vi "button painter (SubVI).vi"(9 "Off state":cluster{"accent color":u32, "accent color":u32}, 10 "On state":T1, 11 "Button ref in":refnum<vi>) -> ()   [LabVIEW 2021]
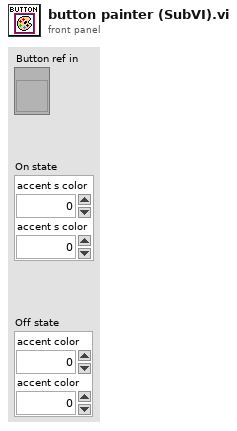
[diagram p1: front panel]
types:
  T1 = cluster{"accent s color":u32, "accent s color":u32}
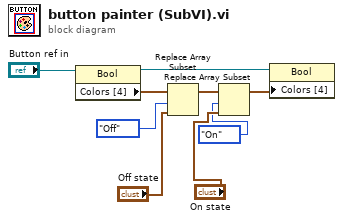
[diagram p0: block diagram]
diagram:
  n1 = property class="Bool"(reference="Button ref in") -> (reference out=w3:refnum<vi>, "Colors [4]"=w2:cluster{u32, u32}[])  [unwired: 1 in, 1 out]
  n2 = Replace Array Subset(array=w2, new element="Off state", index=enum16{"Off", "On"}."Off") -> (w5:cluster{u32, u32}[])
  n3 = Replace Array Subset(array=w5, new element="On state", index=enum16{"Off", "On"}."On") -> (w6:cluster{u32, u32}[])
  n4 = property class="Bool"(reference=w3, "Colors [4]"=w6) -> ()  [unwired: 1 in, 2 out]
